vi "setPort.vi"(10 "Port":u8, 11 "RTDisplacement in":refnum<class "RTDisplacement.lvclass">) -> (3 "RTDisplacement out":refnum<class "RTDisplacement.lvclass">)   [LabVIEW 2016, in "RTDisplacement.lvlib" / "RTDisplacement.lvclass"]
uses:
  RTDisplacement.lvclass
  RTDisplacement.lvclass/RTDisplacement.ctl
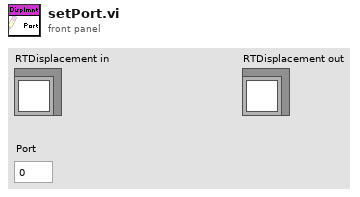
[diagram p1: front panel]
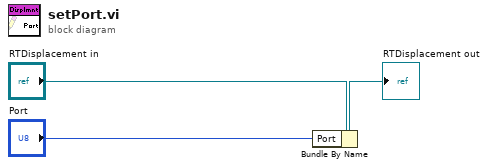
[diagram p0: block diagram]
diagram:
  n1 = Bundle By Name(cluster="RTDisplacement in", "Port"="Port") -> (→"RTDisplacement out":refnum<class "RTDisplacement.lvclass">)
